vi "LIN Kurven anzeigen.vi"() -> ()   [LabVIEW 2020, in "Linearisierung v2.lvlib" / "Protokoll.lvlib"]
uses:
  Protokoll.lvlib
  Visualisierungs Elemente/Button.ctl
  Seiten/FT-IR/FGV FT-IR Gasliste Aktionen.ctl
  Messdaten/Aktionen FGV Messdaten.ctl
  Seiten/FT-IR/FGV FT-IR Parameter.vi
  Allgemein/allgemeine Sub-VIs.lvlib
  Messdaten/Messdaten.lvlib
  Seiten/Grafik/Grafik.lvlib
  Seiten/FT-IR/FT-IR.lvlib
panel:
  in  "Clear 2":T1 caption="Beenden"
  in  "Clear":T1 caption="Beenden"
  in  "Beenden":T1
  in  "Komponenten":T2 {"Komponente 6" items=["---", "NO (3000) LP 191C", "NO2 (150) LP 191C (1of2)", "NO2 (2000) LP 191C (2of2)", "N2O (300) LP 191C (1of2)", "NH3 (300) LP 191C (1of2)", "NH3 (900,3000) LP 191C (2of2)", "HNCO (400) 191C", "H2O% (30) LP 191C", "Formaldehyde (70,500) LP 191C", "CO2 low% (4) LP 191C (2of2)", "CO2% (20) LP 191C (1of2)", "CO (700) LP 191C (1of3)", "CO% (1) LP 191C (2of3)", "Propylene (1000) LP 191C", "Aromatic HC C7 (500) LP 191C", "Ethylene (1000) LP 191C", "CH4 (250) LP 191C (1of2)", "CH4 (5000) LP 191C (2of2)", "Ethane (1000) LP 191C", "Acetylene (1000) LP 191C", "HNO2 (20) 191C", "MeOH (1000) 191C", "CO% (10) LP 191C (3of3)", "Formic Acid (100) 191C", "SO2 (500) LP 191C", "Acetaldehyde (1000) LP 191C", "COS (100) LP 191C", "1,3 butadiene (100) LP 191C", "Oil as Octane (200) LP 191C", "N2O (1000) LP 191C (2of2)", "Propane (200) LP 191C", "NO2 autorange (2000)", "CO autorange (100000)", "CH4 autorange (5000)", "NH3 autorange (3000)", "NOx autorange (3000)", "HCD (10000)", "NMHCD (10000)", "CO2% autorange (20)", "H2Oppm (300000)", "N2O autorange (1000)", "NMNEHCD (3000)", "Temp. Messzelle", "Druck Messzelle", "sBeam@2500", "Temp. HL zu FT-IR", "Temp. HL Extern SP1", "Austrittstemp. FT-IR", "Temp. Schaltschrank", "Konstant 0", "Konstant 50", "Konstant 100", "AK DUMMY"]; "Komponente 5" items=["---", "NO (3000) LP 191C", "NO2 (150) LP 191C (1of2)", "NO2 (2000) LP 191C (2of2)", "N2O (300) LP 191C (1of2)", "NH3 (300) LP 191C (1of2)", "NH3 (900,3000) LP 191C (2of2)", "HNCO (400) 191C", "H2O% (30) LP 191C", "Formaldehyde (70,500) LP 191C", "CO2 low% (4) LP 191C (2of2)", "CO2% (20) LP 191C (1of2)", "CO (700) LP 191C (1of3)", "CO% (1) LP 191C (2of3)", "Propylene (1000) LP 191C", "Aromatic HC C7 (500) LP 191C", "Ethylene (1000) LP 191C", "CH4 (250) LP 191C (1of2)", "CH4 (5000) LP 191C (2of2)", "Ethane (1000) LP 191C", "Acetylene (1000) LP 191C", "HNO2 (20) 191C", "MeOH (1000) 191C", "CO% (10) LP 191C (3of3)", "Formic Acid (100) 191C", "SO2 (500) LP 191C", "Acetaldehyde (1000) LP 191C", "COS (100) LP 191C", "1,3 butadiene (100) LP 191C", "Oil as Octane (200) LP 191C", "N2O (1000) LP 191C (2of2)", "Propane (200) LP 191C", "NO2 autorange (2000)", "CO autorange (100000)", "CH4 autorange (5000)", "NH3 autorange (3000)", "NOx autorange (3000)", "HCD (10000)", "NMHCD (10000)", "CO2% autorange (20)", "H2Oppm (300000)", "N2O autorange (1000)", "NMNEHCD (3000)", "Temp. Messzelle", "Druck Messzelle", "sBeam@2500", "Temp. HL zu FT-IR", "Temp. HL Extern SP1", "Austrittstemp. FT-IR", "Temp. Schaltschrank", "Konstant 0", "Konstant 50", "Konstant 100", "AK DUMMY"]; "Komponente 4" items=["---", "NO (3000) LP 191C", "NO2 (150) LP 191C (1of2)", "NO2 (2000) LP 191C (2of2)", "N2O (300) LP 191C (1of2)", "NH3 (300) LP 191C (1of2)", "NH3 (900,3000) LP 191C (2of2)", "HNCO (400) 191C", "H2O% (30) LP 191C", "Formaldehyde (70,500) LP 191C", "CO2 low% (4) LP 191C (2of2)", "CO2% (20) LP 191C (1of2)", "CO (700) LP 191C (1of3)", "CO% (1) LP 191C (2of3)", "Propylene (1000) LP 191C", "Aromatic HC C7 (500) LP 191C", "Ethylene (1000) LP 191C", "CH4 (250) LP 191C (1of2)", "CH4 (5000) LP 191C (2of2)", "Ethane (1000) LP 191C", "Acetylene (1000) LP 191C", "HNO2 (20) 191C", "MeOH (1000) 191C", "CO% (10) LP 191C (3of3)", "Formic Acid (100) 191C", "SO2 (500) LP 191C", "Acetaldehyde (1000) LP 191C", "COS (100) LP 191C", "1,3 butadiene (100) LP 191C", "Oil as Octane (200) LP 191C", "N2O (1000) LP 191C (2of2)", "Propane (200) LP 191C", "NO2 autorange (2000)", "CO autorange (100000)", "CH4 autorange (5000)", "NH3 autorange (3000)", "NOx autorange (3000)", "HCD (10000)", "NMHCD (10000)", "CO2% autorange (20)", "H2Oppm (300000)", "N2O autorange (1000)", "NMNEHCD (3000)", "Temp. Messzelle", "Druck Messzelle", "sBeam@2500", "Temp. HL zu FT-IR", "Temp. HL Extern SP1", "Austrittstemp. FT-IR", "Temp. Schaltschrank", "Konstant 0", "Konstant 50", "Konstant 100", "AK DUMMY"]; "Komponente 3" items=["---", "NO (3000) LP 191C", "NO2 (150) LP 191C (1of2)", "NO2 (2000) LP 191C (2of2)", "N2O (300) LP 191C (1of2)", "NH3 (300) LP 191C (1of2)", "NH3 (900,3000) LP 191C (2of2)", "HNCO (400) 191C", "H2O% (30) LP 191C", "Formaldehyde (70,500) LP 191C", "CO2 low% (4) LP 191C (2of2)", "CO2% (20) LP 191C (1of2)", "CO (700) LP 191C (1of3)", "CO% (1) LP 191C (2of3)", "Propylene (1000) LP 191C", "Aromatic HC C7 (500) LP 191C", "Ethylene (1000) LP 191C", "CH4 (250) LP 191C (1of2)", "CH4 (5000) LP 191C (2of2)", "Ethane (1000) LP 191C", "Acetylene (1000) LP 191C", "HNO2 (20) 191C", "MeOH (1000) 191C", "CO% (10) LP 191C (3of3)", "Formic Acid (100) 191C", "SO2 (500) LP 191C", "Acetaldehyde (1000) LP 191C", "COS (100) LP 191C", "1,3 butadiene (100) LP 191C", "Oil as Octane (200) LP 191C", "N2O (1000) LP 191C (2of2)", "Propane (200) LP 191C", "NO2 autorange (2000)", "CO autorange (100000)", "CH4 autorange (5000)", "NH3 autorange (3000)", "NOx autorange (3000)", "HCD (10000)", "NMHCD (10000)", "CO2% autorange (20)", "H2Oppm (300000)", "N2O autorange (1000)", "NMNEHCD (3000)", "Temp. Messzelle", "Druck Messzelle", "sBeam@2500", "Temp. HL zu FT-IR", "Temp. HL Extern SP1", "Austrittstemp. FT-IR", "Temp. Schaltschrank", "Konstant 0", "Konstant 50", "Konstant 100", "AK DUMMY"]; "Komponente 2" items=["---", "NO (3000) LP 191C", "NO2 (150) LP 191C (1of2)", "NO2 (2000) LP 191C (2of2)", "N2O (300) LP 191C (1of2)", "NH3 (300) LP 191C (1of2)", "NH3 (900,3000) LP 191C (2of2)", "HNCO (400) 191C", "H2O% (30) LP 191C", "Formaldehyde (70,500) LP 191C", "CO2 low% (4) LP 191C (2of2)", "CO2% (20) LP 191C (1of2)", "CO (700) LP 191C (1of3)", "CO% (1) LP 191C (2of3)", "Propylene (1000) LP 191C", "Aromatic HC C7 (500) LP 191C", "Ethylene (1000) LP 191C", "CH4 (250) LP 191C (1of2)", "CH4 (5000) LP 191C (2of2)", "Ethane (1000) LP 191C", "Acetylene (1000) LP 191C", "HNO2 (20) 191C", "MeOH (1000) 191C", "CO% (10) LP 191C (3of3)", "Formic Acid (100) 191C", "SO2 (500) LP 191C", "Acetaldehyde (1000) LP 191C", "COS (100) LP 191C", "1,3 butadiene (100) LP 191C", "Oil as Octane (200) LP 191C", "N2O (1000) LP 191C (2of2)", "Propane (200) LP 191C", "NO2 autorange (2000)", "CO autorange (100000)", "CH4 autorange (5000)", "NH3 autorange (3000)", "NOx autorange (3000)", "HCD (10000)", "NMHCD (10000)", "CO2% autorange (20)", "H2Oppm (300000)", "N2O autorange (1000)", "NMNEHCD (3000)", "Temp. Messzelle", "Druck Messzelle", "sBeam@2500", "Temp. HL zu FT-IR", "Temp. HL Extern SP1", "Austrittstemp. FT-IR", "Temp. Schaltschrank", "Konstant 0", "Konstant 50", "Konstant 100", "AK DUMMY"]; "Komponente 1" items=["---", "NO (3000) LP 191C", "NO2 (150) LP 191C (1of2)", "NO2 (2000) LP 191C (2of2)", "N2O (300) LP 191C (1of2)", "NH3 (300) LP 191C (1of2)", "NH3 (900,3000) LP 191C (2of2)", "HNCO (400) 191C", "H2O% (30) LP 191C", "Formaldehyde (70,500) LP 191C", "CO2 low% (4) LP 191C (2of2)", "CO2% (20) LP 191C (1of2)", "CO (700) LP 191C (1of3)", "CO% (1) LP 191C (2of3)", "Propylene (1000) LP 191C", "Aromatic HC C7 (500) LP 191C", "Ethylene (1000) LP 191C", "CH4 (250) LP 191C (1of2)", "CH4 (5000) LP 191C (2of2)", "Ethane (1000) LP 191C", "Acetylene (1000) LP 191C", "HNO2 (20) 191C", "MeOH (1000) 191C", "CO% (10) LP 191C (3of3)", "Formic Acid (100) 191C", "SO2 (500) LP 191C", "Acetaldehyde (1000) LP 191C", "COS (100) LP 191C", "1,3 butadiene (100) LP 191C", "Oil as Octane (200) LP 191C", "N2O (1000) LP 191C (2of2)", "Propane (200) LP 191C", "NO2 autorange (2000)", "CO autorange (100000)", "CH4 autorange (5000)", "NH3 autorange (3000)", "NOx autorange (3000)", "HCD (10000)", "NMHCD (10000)", "CO2% autorange (20)", "H2Oppm (300000)", "N2O autorange (1000)", "NMNEHCD (3000)", "Temp. Messzelle", "Druck Messzelle", "sBeam@2500", "Temp. HL zu FT-IR", "Temp. HL Extern SP1", "Austrittstemp. FT-IR", "Temp. Schaltschrank", "Konstant 0", "Konstant 50", "Konstant 100", "AK DUMMY"]}
  out "Grafik":waveform(dbl)[](graph)
  # "Grafik"
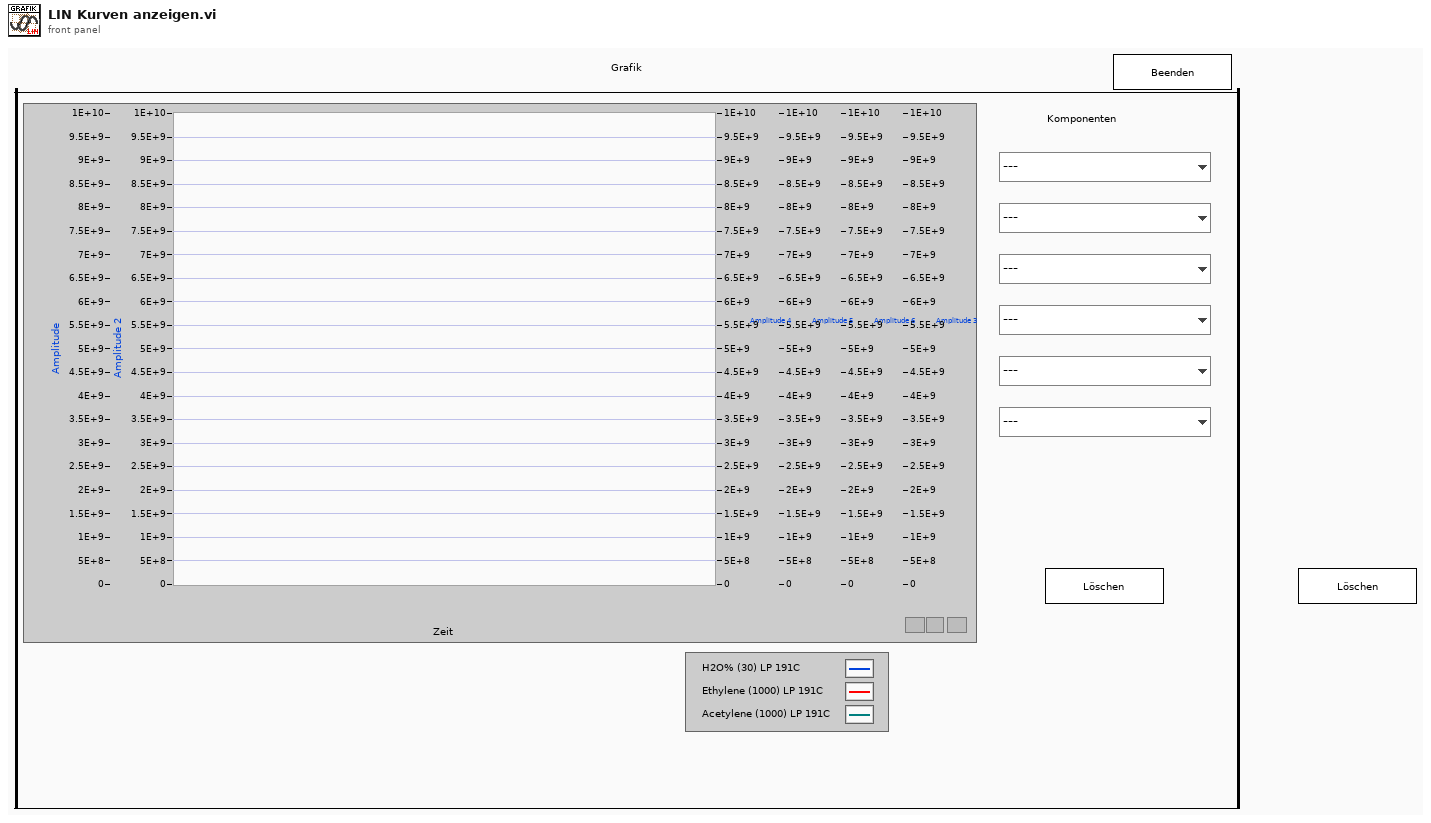
[diagram p1: front panel]
types:
  T1 = typedef "Button.ctl" = bool
  T2 = cluster{"Komponente 1":u16, "Komponente 2":u16, "Komponente 3":u16, "Komponente 4":u16, "Komponente 5":u16, "Komponente 6":u16}
  T3 = typedef "FT-IR.lvlib/FGV FT-IR Gasliste Aktionen.ctl" = enum16{"lesen", "Gasliste FT-IR", "Gasliste ausgelesen", "laden", "speichern", "löschen"}
  T4 = typedef "String - Ausgabefeld.ctl" = string
  T5 = cluster{"Dieses VI":refnum<vi>, "Komponenten":refnum<vi>, "Grafik":refnum<vi>, "Clear":refnum<vi>}
  T6 = typedef "Messdaten.lvlib/Aktionen FGV Messdaten.ctl" = enum16{"lesen", "schreiben", "löschen", "Mittelwerte", "Komponente"}
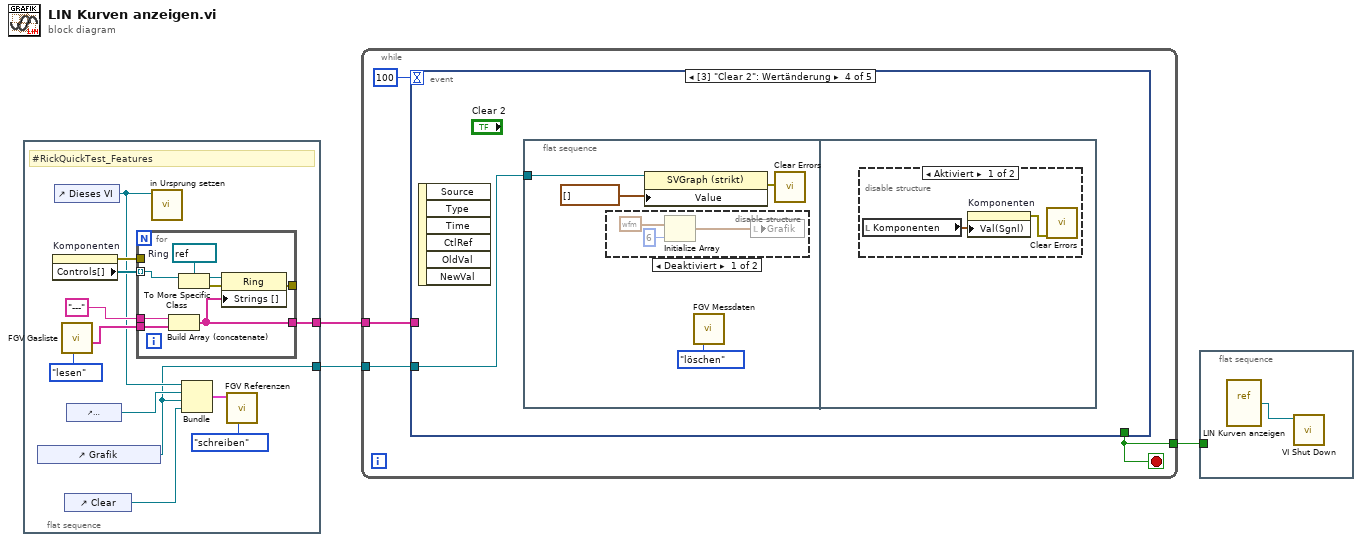
[diagram p0: block diagram]
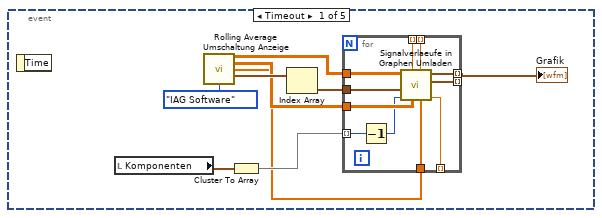
[diagram p2: hidden frame]
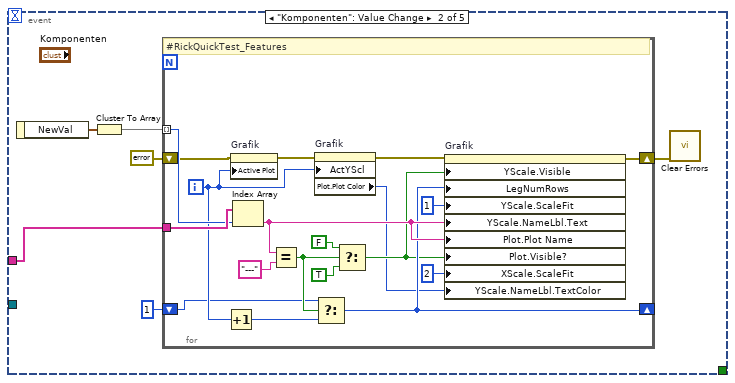
[diagram p3: hidden frame]
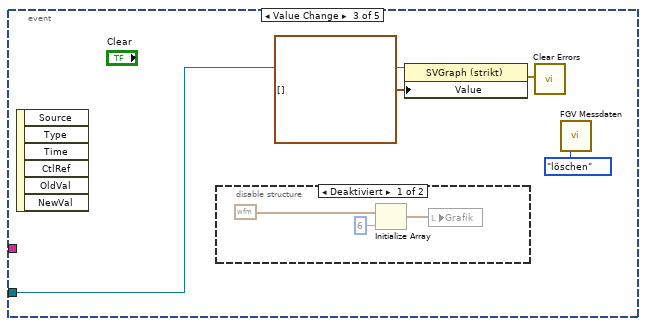
[diagram p4: hidden frame]
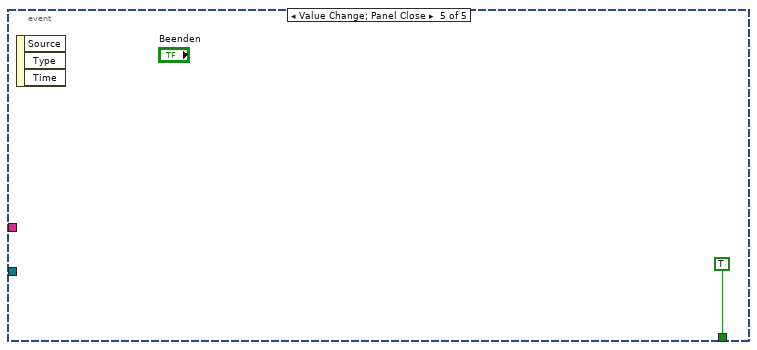
[diagram p8: hidden frame]
diagram:
  n1 = flat-sequence {
    tunnel: [w6] -> w2
    tunnel: [w4] -> w1
    frame #0 {
      # "#RickQuickTest_Features"
      n2 = control-ref of="Grafik"() -> (w4:refnum<vi>)
      n3 = property on="Komponenten" class="Cluster (strikt)"() -> (error out=w11:errorcluster, "Controls[]"=w12:refnum<vi>[])  [unwired: 2 in, 1 out]
      n4 = control-ref of="Dieses VI"() -> (w9:refnum<vi>)
      n5 = call "FGV Gasliste.vi"("Aktionen"=FGV_FT-IR_Gasliste_Aktionen."lesen") -> ("Aktuelle Gasliste gesamt"=w13:T4[])  [unwired: 8 in, 2 out]
      n6 = control-ref of="Clear"() -> (w7:refnum<vi>)
      n7 = control-ref of="Komponenten"() -> (w8:refnum<vi>)
      n8 = for {
        tunnel: "---" ("String") -> [w22]
        tunnel: w13 -> [w21]
        tunnel: w12 -> [w20] mode=indexing
        tunnel: w11 -> [_]
        tunnel: [w17] -> _
        tunnel: [w16] -> w6
        w23 = refnum<vi> refnum  # Ring
        n9 = Build Array (concatenate)(w22, w21) -> (w16:T4[])
        n10 = To More Specific Class(target class=w23, reference=w20) -> (specific class reference=w19:refnum<vi>, error out=w18:errorcluster)  [unwired: 1 in]
        n11 = property class="Ring"(reference=w19, error in=w18, "Strings []"=w16) -> (error out=w17:errorcluster)  [unwired: 1 out]
      }
      n12 = call "in Ursprung setzen.vi"("VI Referenz"=w9) -> ()  [unwired: 10 in, 1 out]
      n13 = Bundle("Dieses VI"=w9, "Komponenten"=w8, "Grafik"=w4, "Clear"=w7) -> (w5:T5)  [unwired: 1 in]
      n14 = call "FGV Referenzen.vi"("Aktikon"=enum16{"lesen", "schreiben"}."schreiben", "Referenzen Cluster in"=w5) -> ()  [unwired: 7 in, 2 out]
    }
  }
  n15 = while {
    tunnel: w2 -> [w26]
    tunnel: [w25] -> w3
    tunnel: w1 -> [w24]
    stop <- w25 stop-if-true
    n16 = event shown="[3] \"Clear 2\": Wertänderung" {
      selector: _ -> [_ _ _ _ _]
      dyn-events: _ -> [_ _ _ _ _]
      timeout: 100 -> [_ _ _ _ _]
      tunnel: [_ _ _ _ TRUE] -> w25
      tunnel: w26 -> [_ w51 _ _ _]
      tunnel: w24 -> [_ _ w76 w80 _]
      event Timeout {
        n17 = event-data() -> ()  [unwired: 1 in, 1 out]
        n18 = local read "Komponenten"() -> (w34:T2)
        n19 = call "Rolling Average Umschaltung Anzeige.vi"("Aktion"=enum16{"AK", "IAG Software"}."IAG Software") -> ("Messdaten"=w31:sgl[][], "Mittelwertdaten"=w30:sgl[][], "Deviation"=w29:sgl[], "Zeitstempeln"=w35:timestamp[])  [unwired: 9 in, 2 out]
        n20 = Cluster To Array(cluster=w34) -> (array=w32:u16[])
        n21 = Index Array(array=w35) -> (element=w33:timestamp)  [unwired: 1 in]
        n22 = for {
          tunnel: w32 -> [w47] mode=indexing
          tunnel: w31 -> [w46]
          tunnel: w33 -> [w45]
          tunnel: w30 -> [w38]
          tunnel: w29 -> [w44]
          tunnel: [w43] -> _ mode=indexing
          tunnel: [w42] -> _ mode=indexing
          tunnel: [w41] -> w28 mode=indexing
          tunnel: [w40] -> _ mode=indexing
          tunnel: [w39] -> _ mode=indexing
          n23 = Decrement(x=w47) -> (x-1=w37:u16)
          n24 = call "Signalverlaeufe in Graphen Umladen.vi"("Deviation"=w44, "Mittelwertdaten"=w38, "Gas-Auswahl"=w37, "t0"=w45, "Werte"=w46) -> ("Konzentration"=w43:sgl, "Mittelwert"=w42:waveform(dbl), "Waveform"=w41:waveform(dbl), "aktuelle Mittelwert"=w40:sgl, "Deviation"=w39:sgl)  [unwired: 2 in]
        }
        "Grafik" <- w28
      }
      event "Komponenten": Value Change {
        n25 = event-data() -> ("NewVal"=w53:T2)  [unwired: 1 in]
        n26 = Cluster To Array(cluster=w53) -> (array=w52:u16[])
        n27 = for {
          tunnel: w52 -> [w64] mode=indexing
          tunnel: w51 -> [w68]
          shift-right: [w58] -> _
          shift-left: 1 -> [w60]
          shift-right: [w72] -> w48
          shift-left: errorcluster {"status"=FALSE, "code"=0, "source"=""} ("Fehler (Ausgang)") -> [w55]
          i -> [w61]
          # "#RickQuickTest_Features"
          n28 = Increment(x=w61) -> (x+1=w59:i32)
          n29 = property on="Grafik" class="SVGraph (strikt)"(error in=w55, "Active Plot"=w61) -> (error out=w71:errorcluster)  [unwired: 1 in, 1 out]
          n30 = Index Array(array=w68, index=w64) -> (element=w65:T4)
          n31 = Equal?(x=w65, y="---" ("String")) -> (x = y?=w62:bool)
          n32 = property on="Grafik" class="SVGraph (strikt)"(error in=w71, "ActYScl"=w61) -> (error out=w70:errorcluster, "Plot.Plot Color"=w54:u32)  [unwired: 1 in, 1 out]
          n33 = Select(t=w60, s=w62, f=w59) -> (s? t:f=w58:i32)
          n34 = Select(t=FALSE, s=w62, f=TRUE) -> (s? t:f=w57:bool)
          n35 = property on="Grafik" class="SVGraph (strikt)"(error in=w70, "YScale.Visible"=w57, "LegNumRows"=w58, "YScale.ScaleFit"=u8 1 ("Y-Achse.Achsenanpassung"), "YScale.NameLbl.Text"=w65, "Plot.Plot Name"=w65, "Plot.Visible?"=w57, "XScale.ScaleFit"=u8 2 ("X-Achse.Achsenanpassung"), "YScale.NameLbl.TextColor"=w54) -> (error out=w72:errorcluster)  [unwired: 1 in, 1 out]
        }
        n36 = call <vilib>:"Clear Errors.vi"("error in (no error)"=w48) -> ()  [unwired: 5 in, 2 out]
      }
      event Value Change {
        n37 = event-data() -> ()  [unwired: 1 in, 6 out]
        n38 = disable-structure shown="Deaktiviert" {
          frame Disabled {
            n39 = Initialize Array(waveform(dbl) {"t0"=timestamp(0 s since 1904-01-01), "dt"=1.0, "Y"=[]} ("Waveform"), 6 ("Dimensionsgröße")) -> (w77:waveform(dbl)[])
            n40 = local write "Grafik"(w77) -> ()
          }
          frame Enabled {
          }
        }
        n41 = property class="SVGraph (strikt)"(reference=w76, "Value"=waveform(dbl)[] [] ("Wert")) -> (error out=w75:errorcluster)  [unwired: 1 in, 1 out]
        n42 = call <vilib>:"Clear Errors.vi"("error in (no error)"=w75) -> ()  [unwired: 5 in, 2 out]
        n43 = call "FGV Messdaten.vi"("Aktionen"=Aktionen_FGV_Messdaten."löschen") -> ()  [unwired: 6 in, 9 out]
      }
      event Value Change {
        n44 = event-data() -> ()  [unwired: 1 in, 6 out]
        n45 = flat-sequence {
          tunnel: w80 -> [w84]
          frame #0 {
            n46 = disable-structure shown="Deaktiviert" {
              frame Disabled {
                n47 = Initialize Array(waveform(dbl) {"t0"=timestamp(0 s since 1904-01-01), "dt"=1.0, "Y"=[]} ("Waveform"), 6 ("Dimensionsgröße")) -> (w85:waveform(dbl)[])
                n48 = local write "Grafik"(w85) -> ()
              }
              frame Enabled {
              }
            }
            n49 = property class="SVGraph (strikt)"(reference=w84, "Value"=waveform(dbl)[] [] ("Wert")) -> (error out=w83:errorcluster)  [unwired: 1 in, 1 out]
            n50 = call "FGV Messdaten.vi"("Aktionen"=Aktionen_FGV_Messdaten."löschen") -> ()  [unwired: 6 in, 9 out]
            n51 = call <vilib>:"Clear Errors.vi"("error in (no error)"=w83) -> ()  [unwired: 5 in, 2 out]
          }
          frame #1 {
            n52 = disable-structure shown="Aktiviert" {
              frame Enabled {
                n53 = local read "Komponenten"() -> (w89:T2)
                n54 = property on="Komponenten" class="Cluster (strikt)"("Val(Sgnl)"=w89) -> (error out=w88:errorcluster)  [unwired: 2 in, 1 out]
                n55 = call <vilib>:"Clear Errors.vi"("error in (no error)"=w88) -> ()  [unwired: 5 in, 2 out]
              }
              frame Disabled {
              }
            }
          }
        }
      }
      event Value Change; Panel Close {
        n56 = event-data() -> ()  [unwired: 1 in, 3 out]
      }
    }
  }
  n57 = flat-sequence {
    tunnel: w3 -> [_]
    frame #0 {
      n58 = vi-ref "LIN Kurven anzeigen.vi"() -> (w91:refnum<vi>)
      n59 = call "VI Shut Down.vi"("VI Referenz"=w91) -> ()  [unwired: 11 in]
    }
  }
